vi "GCM_ConfigurationFolder.vi"() -> (3 "ConfigurationFolder":path)   [LabVIEW 2014]
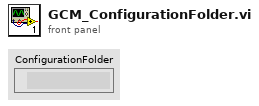
[diagram p1: front panel]
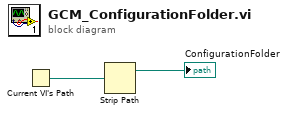
[diagram p0: block diagram]
diagram:
  n1 = Current VI's Path() -> (path=w2:path)
  n2 = Strip Path(path=w2) -> (stripped path=→"ConfigurationFolder":path)  [unwired: 1 out]
